vi "test json to variant enum.vi"(8 "error in (no error)":errorcluster) -> (0 "error out":errorcluster)   [LabVIEW 2019, in "labview_json_tests.lvlib"]
uses:
  labview_json_tests.lvlib
  lib/labview_json.lvlib
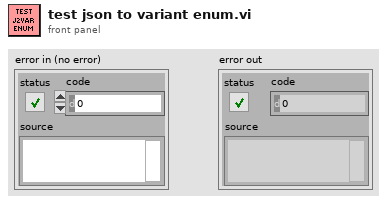
[diagram p1: front panel]
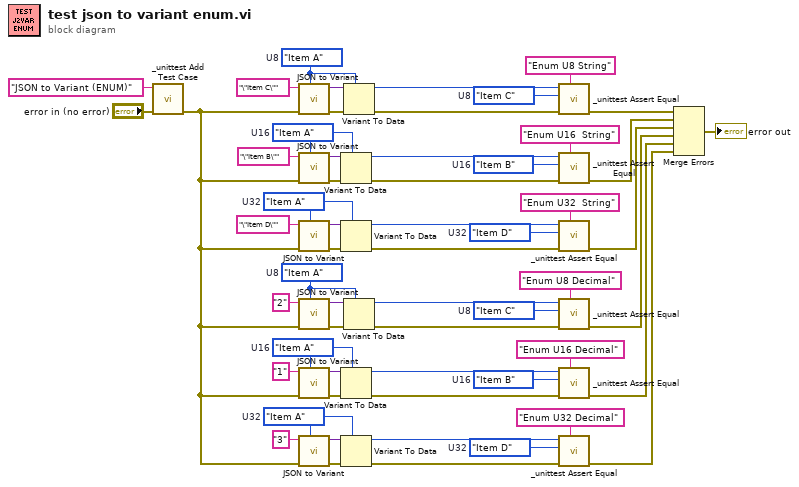
[diagram p0: block diagram]
diagram:
  w28 = enum32{"Item A", "Item B", "Item C", "Item D"}."Item D"  # U32
  w24 = enum16{"Item A", "Item B", "Item C", "Item D"}."Item B"  # U16
  w18 = enum8{"Item A", "Item B", "Item C", "Item D"}."Item C"  # U8
  w25 = enum32{"Item A", "Item B", "Item C", "Item D"}."Item A"  # U32
  w22 = enum16{"Item A", "Item B", "Item C", "Item D"}."Item A"  # U16
  w16 = enum8{"Item A", "Item B", "Item C", "Item D"}."Item A"  # U8
  w29 = enum32{"Item A", "Item B", "Item C", "Item D"}."Item D"  # U32
  w33 = enum16{"Item A", "Item B", "Item C", "Item D"}."Item B"  # U16
  w39 = enum8{"Item A", "Item B", "Item C", "Item D"}."Item C"  # U8
  w32 = enum32{"Item A", "Item B", "Item C", "Item D"}."Item A"  # U32
  w35 = enum16{"Item A", "Item B", "Item C", "Item D"}."Item A"  # U16
  w41 = enum8{"Item A", "Item B", "Item C", "Item D"}."Item A"  # U8
  n1 = call "_unittest Add Test Case.vi"("error in (no error)"="error in (no error)", "Test Case"="JSON to Variant (ENUM)") -> ("error out"=w4:errorcluster)  [unwired: 9 in]
  n2 = call "JSON to Variant.vi"("Variant Type"=w41, "error in (no error)"=w4, "JSON"="\"Item C\"") -> ("error out"=w53:errorcluster, "Variant out"=w42:variant)  [unwired: 7 in]
  n3 = call "JSON to Variant.vi"("Variant Type"=w35, "error in (no error)"=w4, "JSON"="\"Item B\"") -> ("error out"=w50:errorcluster, "Variant out"=w36:variant)  [unwired: 7 in]
  n4 = call "JSON to Variant.vi"("Variant Type"=w32, "error in (no error)"=w4, "JSON"="\"Item D\"") -> ("error out"=w46:errorcluster, "Variant out"=w31:variant)  [unwired: 7 in]
  n5 = call "JSON to Variant.vi"("Variant Type"=w16, "error in (no error)"=w4, "JSON"="2") -> ("error out"=w6:errorcluster, "Variant out"=w15:variant)  [unwired: 7 in]
  n6 = call "JSON to Variant.vi"("Variant Type"=w22, "error in (no error)"=w4, "JSON"="1") -> ("error out"=w9:errorcluster, "Variant out"=w21:variant)  [unwired: 7 in]
  n7 = call "JSON to Variant.vi"("Variant Type"=w25, "error in (no error)"=w4, "JSON"="3") -> ("error out"=w12:errorcluster, "Variant out"=w26:variant)  [unwired: 7 in]
  n8 = Variant To Data(error in=w50, type=w35, Variant=w36) -> (data=w34:enum16{"Item A", "Item B", "Item C", "Item D"}, error out=w38:errorcluster)
  n9 = Variant To Data(error in=w46, type=w32, Variant=w31) -> (data=w30:enum32{"Item A", "Item B", "Item C", "Item D"}, error out=w37:errorcluster)
  n10 = Variant To Data(error in=w9, type=w22, Variant=w21) -> (data=w23:enum16{"Item A", "Item B", "Item C", "Item D"}, error out=w19:errorcluster)
  n11 = Variant To Data(error in=w12, type=w25, Variant=w26) -> (data=w27:enum32{"Item A", "Item B", "Item C", "Item D"}, error out=w20:errorcluster)
  n12 = Variant To Data(error in=w53, type=w41, Variant=w42) -> (data=w40:enum8{"Item A", "Item B", "Item C", "Item D"}, error out=w43:errorcluster)
  n13 = Variant To Data(error in=w6, type=w16, Variant=w15) -> (data=w17:enum8{"Item A", "Item B", "Item C", "Item D"}, error out=w14:errorcluster)
  n14 = call "_unittest Assert Equal.vi"("Message"="Enum U8 String", "error in (no error)"=w43, "Expected Value"=w39, "Actual Value"=w40) -> ("error out"=w56:errorcluster)  [unwired: 7 in]
  n15 = call "_unittest Assert Equal.vi"("Message"="Enum U16  String", "error in (no error)"=w38, "Expected Value"=w33, "Actual Value"=w34) -> ("error out"=w48:errorcluster)  [unwired: 7 in]
  n16 = call "_unittest Assert Equal.vi"("Message"="Enum U32  String", "error in (no error)"=w37, "Expected Value"=w29, "Actual Value"=w30) -> ("error out"=w44:errorcluster)  [unwired: 7 in]
  n17 = call "_unittest Assert Equal.vi"("Message"="Enum U8 Decimal", "error in (no error)"=w14, "Expected Value"=w18, "Actual Value"=w17) -> ("error out"=w3:errorcluster)  [unwired: 7 in]
  n18 = call "_unittest Assert Equal.vi"("Message"="Enum U16 Decimal", "error in (no error)"=w19, "Expected Value"=w24, "Actual Value"=w23) -> ("error out"=w2:errorcluster)  [unwired: 7 in]
  n19 = call "_unittest Assert Equal.vi"("Message"="Enum U32 Decimal", "error in (no error)"=w20, "Expected Value"=w28, "Actual Value"=w27) -> ("error out"=w1:errorcluster)  [unwired: 7 in]
  n20 = Merge Errors(w56, w48, w44, w3, w2, w1) -> (→"error out":errorcluster)
